vi "UT_Kolmogan.vi"() -> ()   [LabVIEW 2019, in "Kolmogan Library 1.lvlib"]
uses:
  Kolmogan Library 1.lvlib
panel:
  out "data out":string
  out "State":i32
  out "current time":timestamp
  out "Result":string
  in  "COGNEX Command":bool
  in  "IP:Port COGNEX Result":string="192.168.0.30"
  in  "IP:Port COGNEX Command":string="192.168.0.30:23"
  out "MS error out":errorcluster
  out "PL.FB error out":errorcluster
  in  "milliseconds to wait":u32=500
  in  "Continue Read":bool
  out "PL.FB":i64
  out "data":bool[](array[boolean])
  in  "RD_DRVMOTIONSTAT":bool
  in  "RD_POSITION_FEEDBACK":bool
  in  "KOLMOGAN指令":u8(ring) items=["0. 復歸", "1. 找原點", "2. 至起始位置", "3. 啟動相機", "4. 掃描拍攝", "SB"]
  out "Error Out":errorcluster
  in  "Error In":errorcluster
  in  "IP:Port":string="192.168.1.11:502"
  in  "Close API":bool
  in  "stop":bool
  in  "Connect PLC":bool
  # "Trigger+Call Motion"
  # "State machine (等待觸發燈號)\n1. 建立連線\n2. 復歸 [ SW(F), Camera(F) ]\n3. 找原點 (Home position found)\n4. 初始位置 (15)\n等待觸發\n>>相機\n>>掃描 (15)\n>>復歸 [ SW(F), Camera(F) ]\nError 重新建立連線"
  # "#588 959/1174 這邊要問Andy"
  # "#268 600/1174 State"
  # "1"
  # "2"
  # "3"
  # "Motion task reach position"
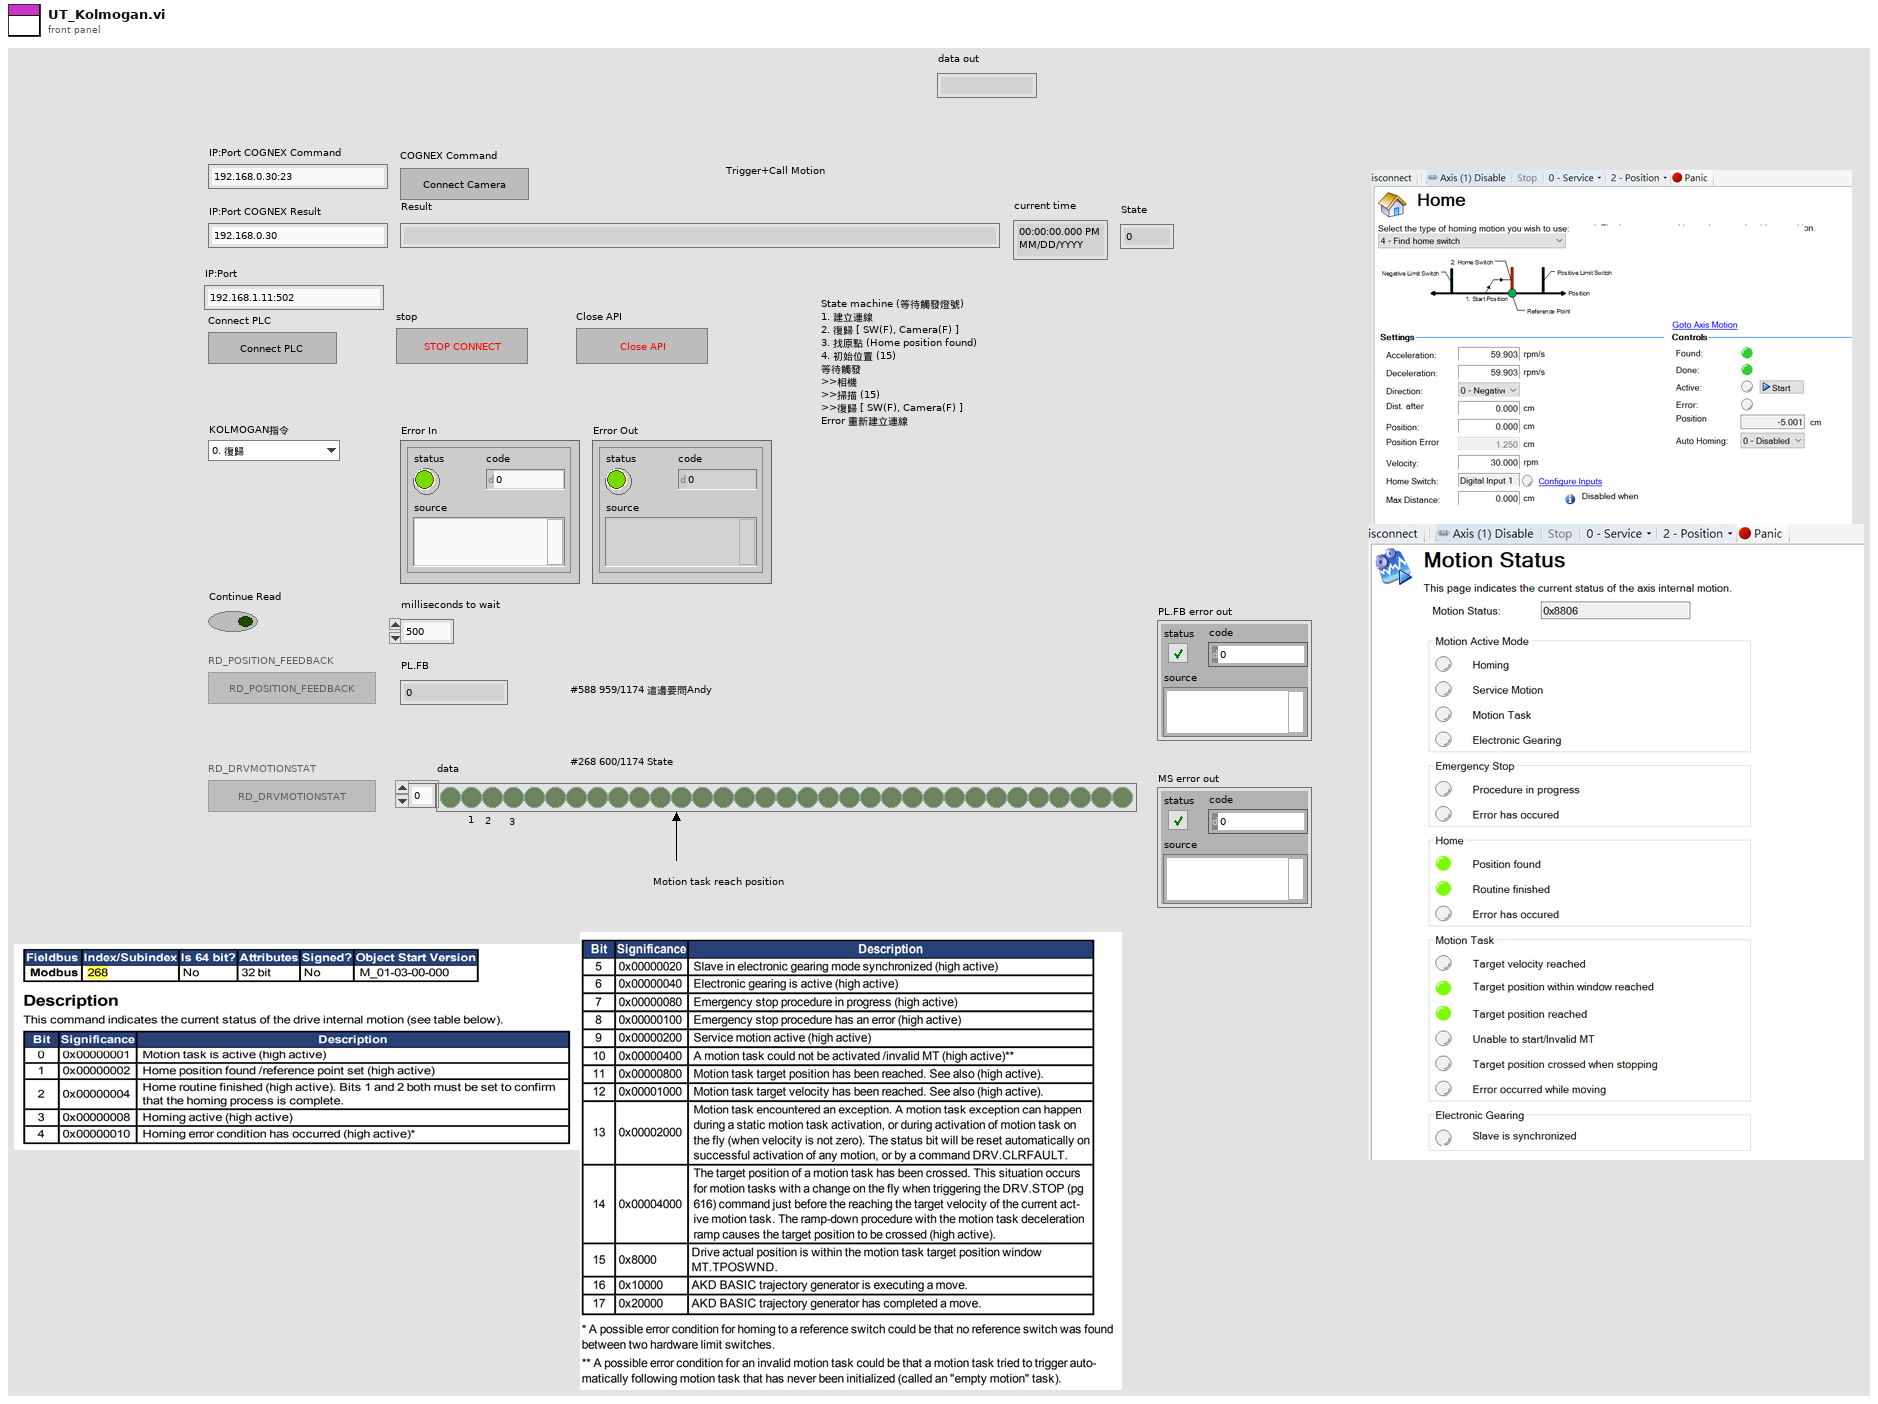
[diagram p1: front panel]
types:
  T1 = enum8{"Enabled", "Disabled", "Disabled and Grayed Out"}
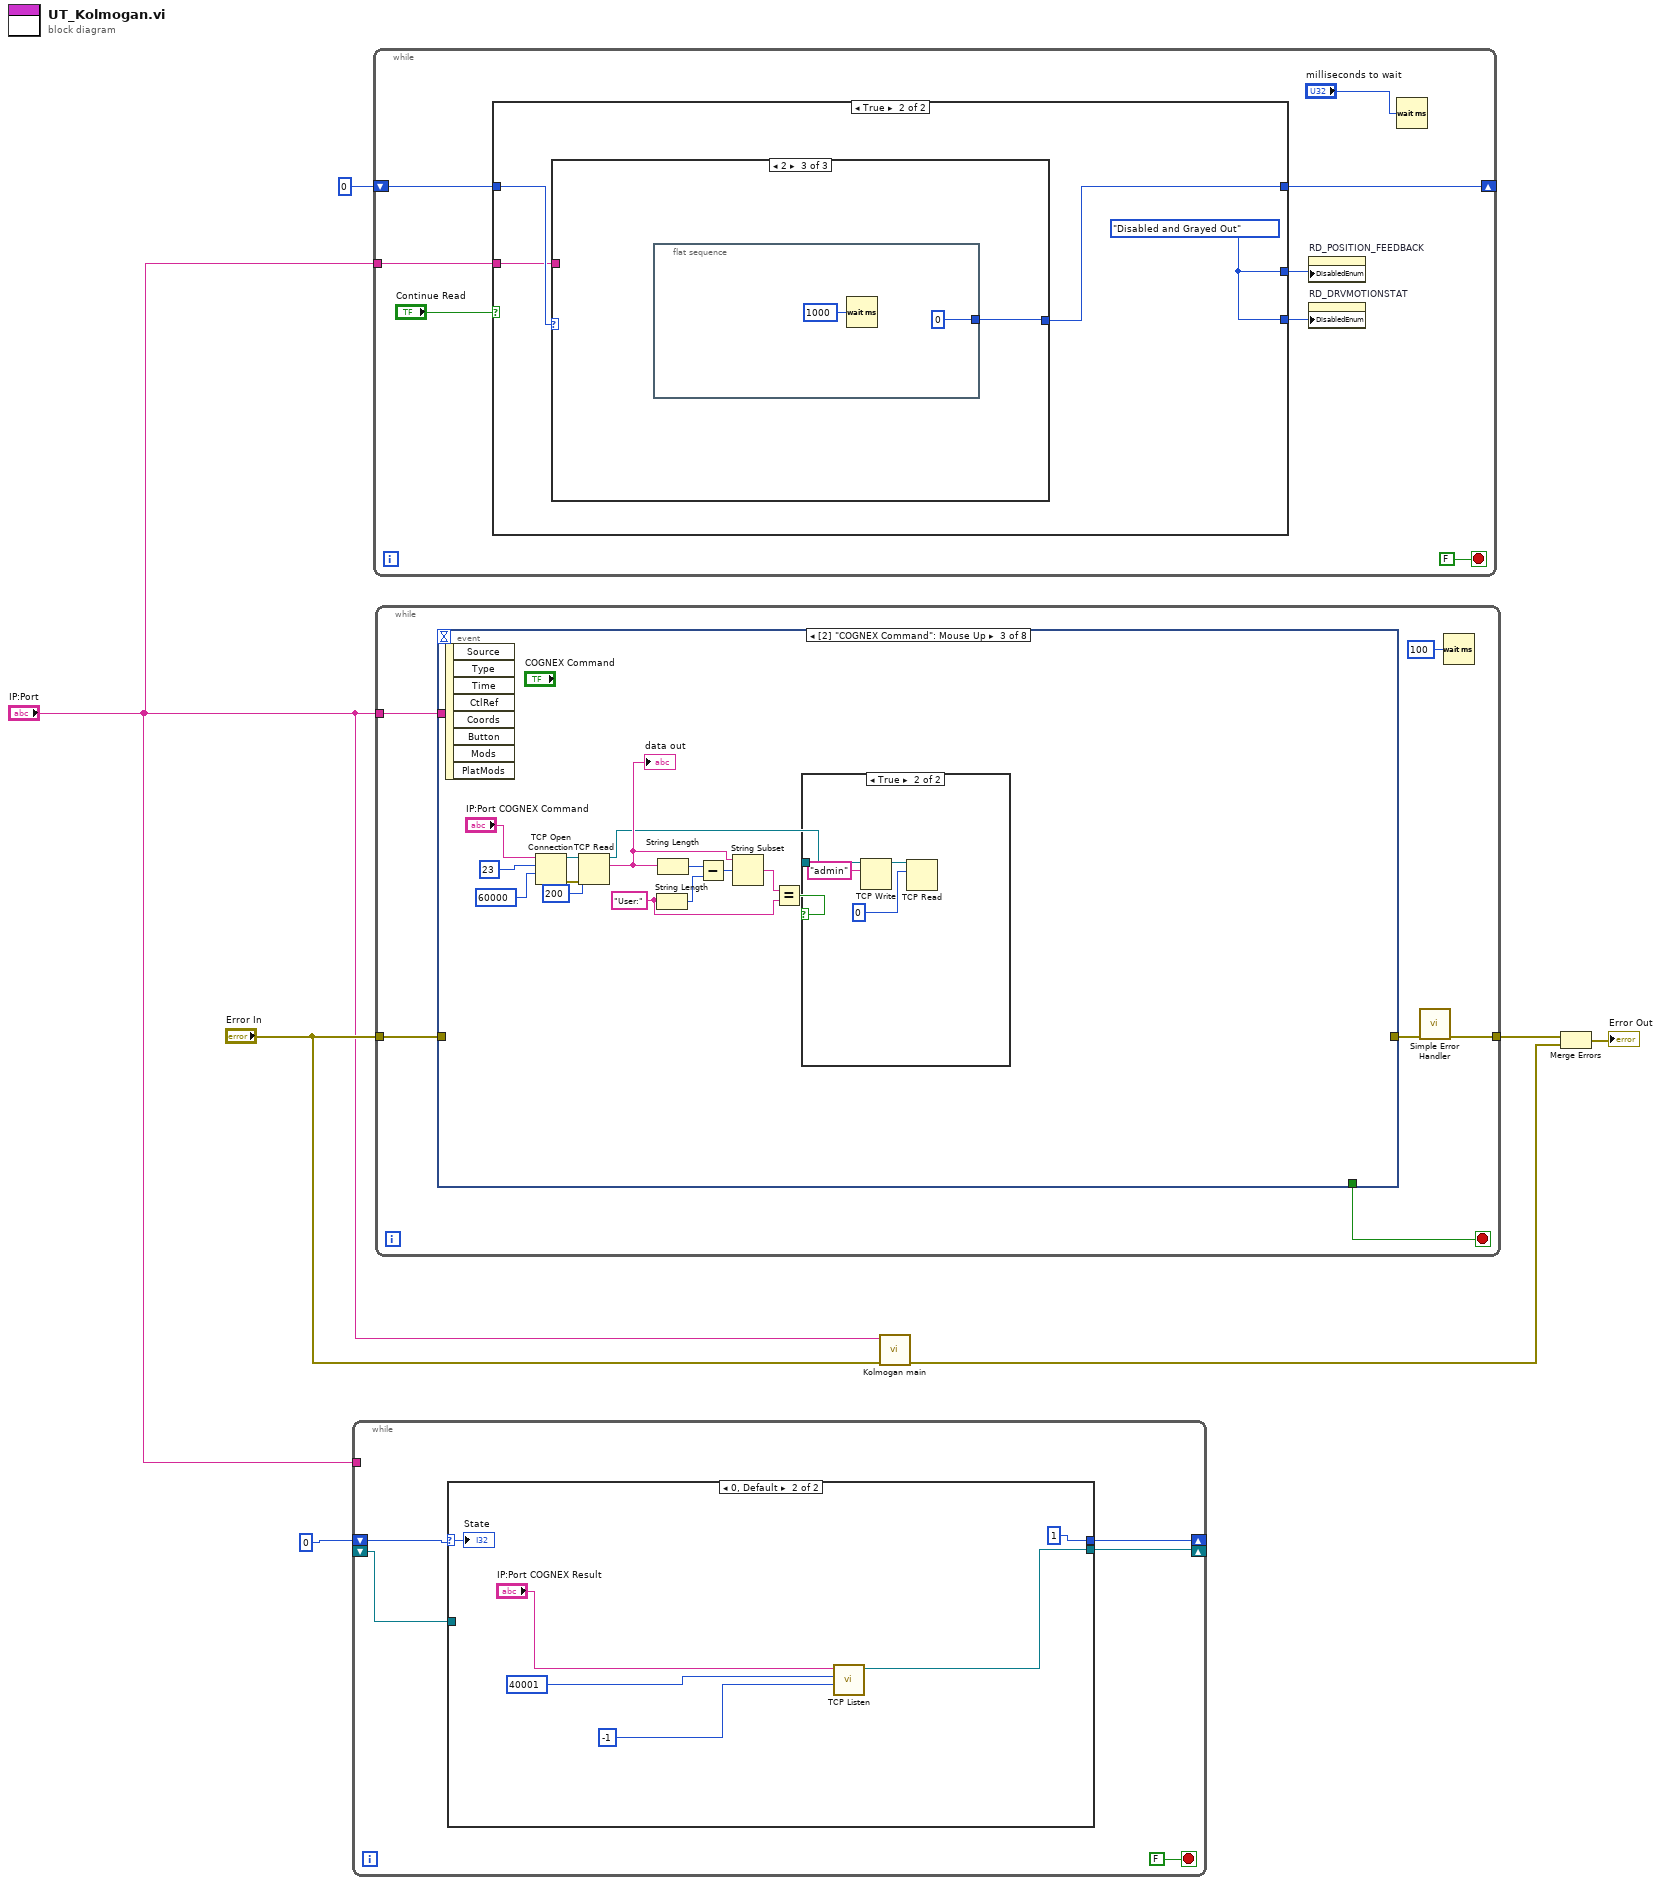
[diagram p0: block diagram]
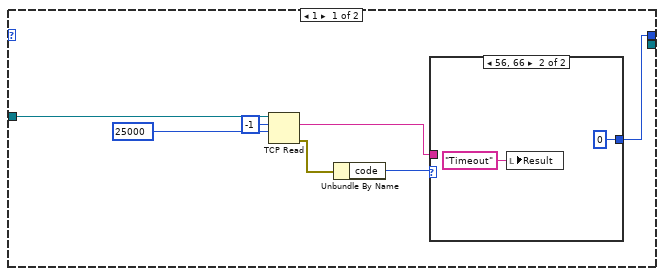
[diagram p2: hidden frame]
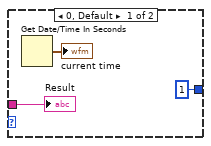
[diagram p3: hidden frame]
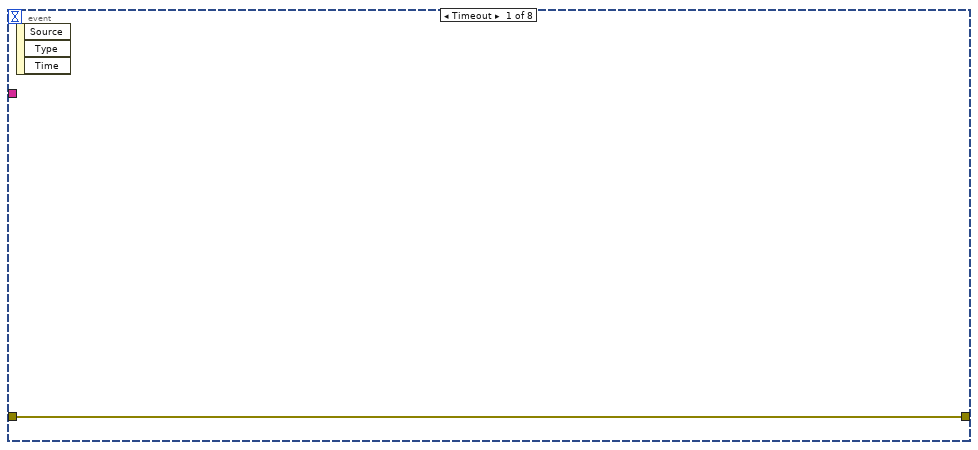
[diagram p4: hidden frame]
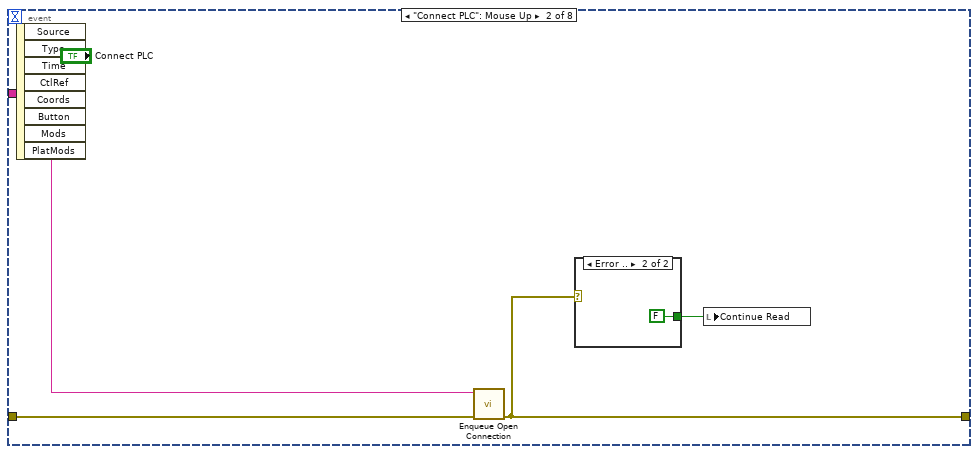
[diagram p5: hidden frame]
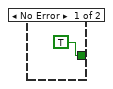
[diagram p6: hidden frame]
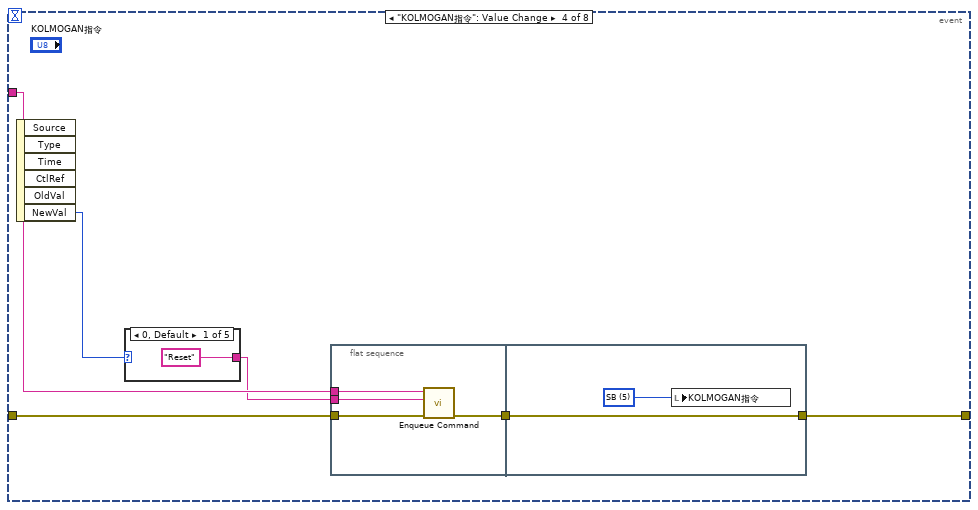
[diagram p8: hidden frame]
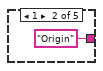
[diagram p9: hidden frame]
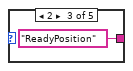
[diagram p10: hidden frame]
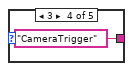
[diagram p11: hidden frame]
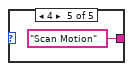
[diagram p12: hidden frame]
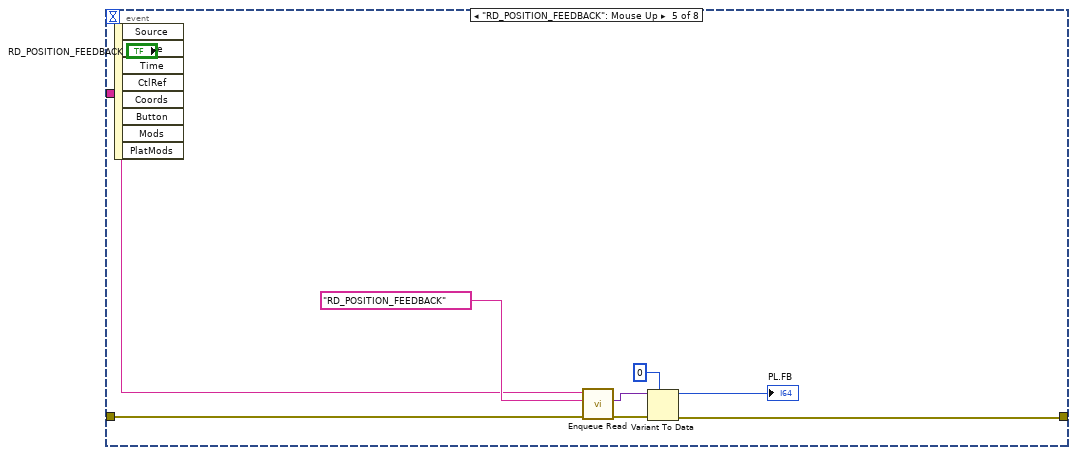
[diagram p13: hidden frame]
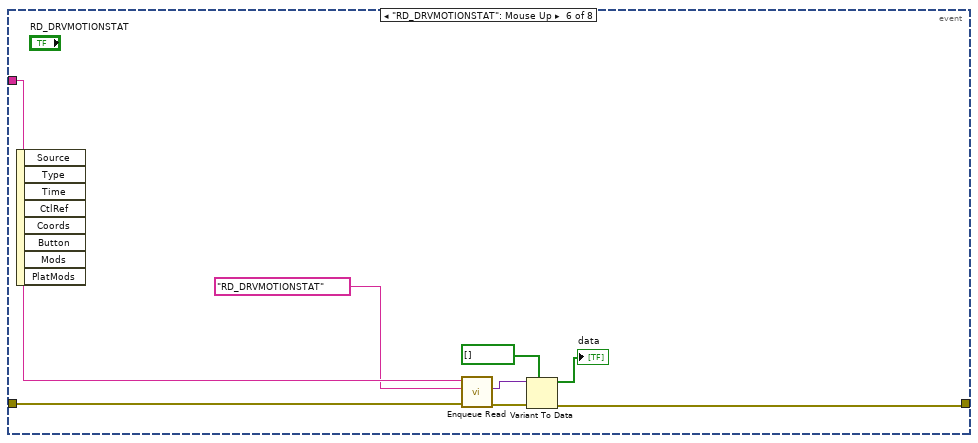
[diagram p14: hidden frame]
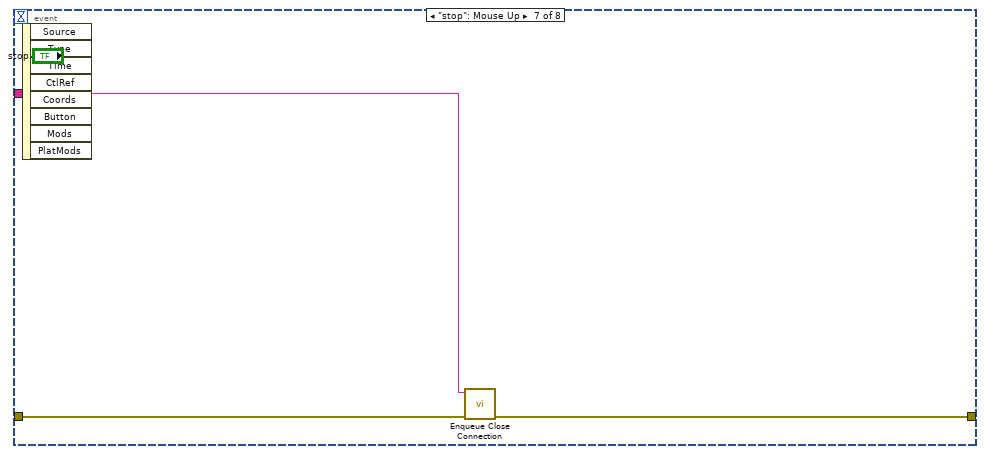
[diagram p15: hidden frame]
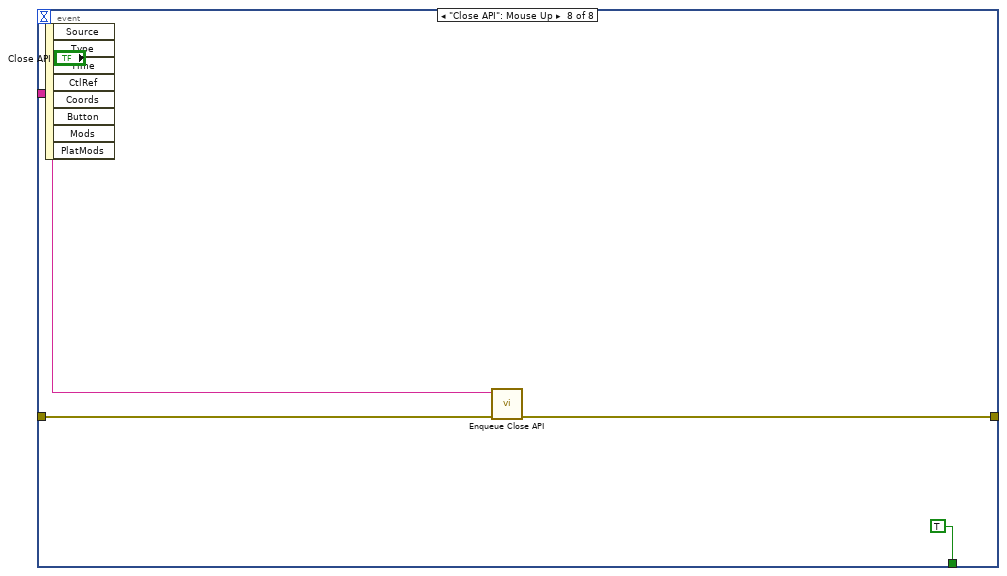
[diagram p16: hidden frame]
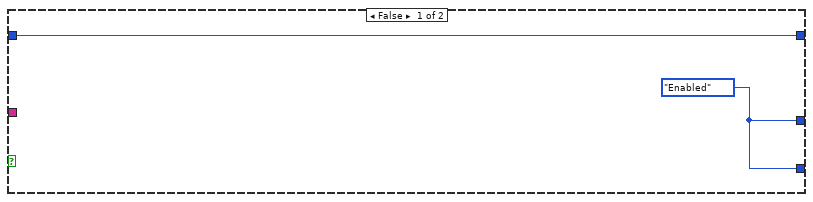
[diagram p17: hidden frame]
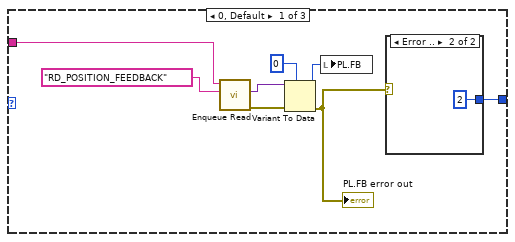
[diagram p18: hidden frame]
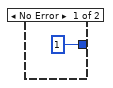
[diagram p19: hidden frame]
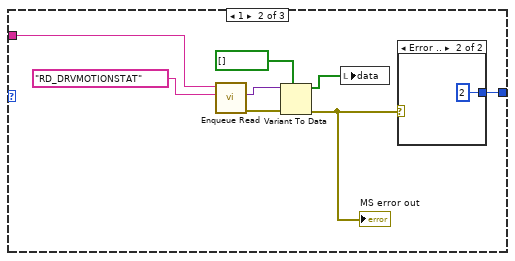
[diagram p20: hidden frame]
diagram:
  n1 = while {
    shift-right: [w11] -> _
    shift-left: _ -> [w8]
    shift-right: [w9] -> _
    shift-left: 0 ("timeout ms (wait forever: -1)") -> [w10]
    tunnel: "IP:Port" -> [_]
    stop <- FALSE stop-if-true
    n2 = case shown="0, Default" w10 {
      selector: w10 -> [_ w25]
      tunnel: [_ w27] -> w11
      tunnel: [w16 1 ("timeout ms (wait forever: -1)")] -> w9
      tunnel: w8 -> [w19 _]
      frame 1 {
        n3 = TCP Read(connection ID=w19, bytes to read=-1, 9:25000 ("timeout ms (25000)")) -> (data out=w13:string, error out=w15:errorcluster)  [unwired: 2 in, 1 out]
        n4 = Unbundle By Name(w15) -> ("code"=w14:i32)
        n5 = case shown="56, 66" w14 {
          tunnel: [1 ("timeout ms (wait forever: -1)") 0 ("timeout ms (wait forever: -1)")] -> w16
          tunnel: w13 -> [w21 _]
          frame 0, Default {
            n6 = Get Date/Time In Seconds() -> (seconds since 1Jan1904=→"current time":timestamp)
            "Result" <- w21
          }
          frame 56, 66 {
            n7 = local write "Result"("Timeout" ("Result")) -> ()
          }
        }
      }
      frame 0, Default {
        n8 = call <vilib>:"TCP Listen.vi"("timeout ms (wait forever: -1)"=-1, "port"=u16 40001, "service name"="IP:Port COGNEX Result") -> ("connection ID"=w27:refnum<k5>)  [unwired: 4 in, 4 out]
        "State" <- w25
      }
    }
  }
  n9 = while {
    tunnel: "IP:Port" -> [w34]
    shift-right: [w33] -> _
    shift-left: 0 -> [w32]
    stop <- FALSE stop-if-true
    n10 = case shown="True" "Continue Read" {
      tunnel: [w40 w44] -> w37
      tunnel: [w40 w44] -> w36
      tunnel: w32 -> [w39 w43]
      tunnel: w34 -> [_ w42]
      tunnel: [w39 w41] -> w33
      frame False {
        w40 = T1."Enabled" ("Disabled")
      }
      frame True {
        w44 = T1."Disabled and Grayed Out" ("Disabled")
        n11 = case shown="2" w43 {
          tunnel: w42 -> [w47 w57 _]
          tunnel: [w46 w56 w65] -> w41
          frame 0, Default {
            n12 = call "Enqueue Read.vi"("Message"="RD_POSITION_FEEDBACK", "Name"=w47) -> ("Error Out"=w50:errorcluster, "Data"=w51:variant)  [unwired: 8 in]
            n13 = Variant To Data(error in=w50, type=i64 0, Variant=w51) -> (data=w52:i64, error out=w45:errorcluster)
            "PL.FB error out" <- w45
            n14 = local write "PL.FB"(w52) -> ()
            n15 = case shown="Error .." w45 {
              tunnel: [1 2] -> w46
              frame No Error {
              }
              frame Error {
              }
            }
          }
          frame 1 {
            n16 = call "Enqueue Read.vi"("Message"="RD_DRVMOTIONSTAT", "Name"=w57) -> ("Error Out"=w60:errorcluster, "Data"=w61:variant)  [unwired: 8 in]
            n17 = Variant To Data(error in=w60, type=bool[] [] ("appended array"), Variant=w61) -> (data=w62:bool[], error out=w55:errorcluster)
            "MS error out" <- w55
            n18 = local write "data"(w62) -> ()
            n19 = case shown="Error .." w55 {
              tunnel: [0 2] -> w56
              frame No Error {
              }
              frame Error {
              }
            }
          }
          frame 2 {
            n20 = flat-sequence {
              tunnel: [0] -> w65
              frame #0 {
                n21 = Wait (ms)(milliseconds to wait=u32 1000) -> ()  [unwired: 1 out]
              }
            }
          }
        }
      }
    }
    n22 = property on="RD_POSITION_FEEDBACK" class="Bool (strict)"("DisabledEnum"=w37) -> ()  [unwired: 2 in, 2 out]
    n23 = property on="RD_DRVMOTIONSTAT" class="Bool (strict)"("DisabledEnum"=w36) -> ()  [unwired: 2 in, 2 out]
    n24 = Wait (ms)(milliseconds to wait="milliseconds to wait") -> ()  [unwired: 1 out]
  }
  n25 = while {
    tunnel: "IP:Port" -> [w73]
    tunnel: "Error In" -> [w72]
    tunnel: [w70] -> w6
    stop <- w69 stop-if-true
    n26 = event shown="[2] \"COGNEX Command\": Mouse Up" {
      selector: _ -> [_ _ _ _ _ _ _ _]
      dyn-events: _ -> [_ _ _ _ _ _ _ _]
      timeout: _ -> [_ _ _ _ _ _ _ _]
      tunnel: w73 -> [_ w77 _ w103 w119 w131 w133 w137]
      tunnel: w72 -> [w74 w78 _ w102 w120 w130 w134 w138]
      tunnel: [w74 w76 _ w101 w117 w126 w132 w136] -> w71
      tunnel: [_ _ _ _ _ _ _ TRUE] -> w69
      event Timeout {
        n27 = event-data() -> ()  [unwired: 1 in, 3 out]
      }
      event "Connect PLC": Mouse Up {
        n28 = event-data() -> ()  [unwired: 1 in, 8 out]
        n29 = call "Enqueue Open Connection.vi"("Error In"=w78, "Name"=w77) -> ("Error Out"=w76:errorcluster)  [unwired: 9 in]
        n30 = case shown="Error .." w76 {
          tunnel: [TRUE ("Continue Read") FALSE ("Continue Read")] -> w75
          frame No Error {
          }
          frame Error {
          }
        }
        n31 = local write "Continue Read"(w75) -> ()
      }
      event "COGNEX Command": Mouse Up {
        w83 = "User:" ("string")
        n32 = event-data() -> ()  [unwired: 1 in, 8 out]
        n33 = TCP Open Connection(address="IP:Port COGNEX Command", remote port or service name=u16 23, timeout ms (60000)=60000) -> (connection ID=w90:refnum<k5>, error out=w91:errorcluster)  [unwired: 2 in]
        n34 = TCP Read(connection ID=w90, bytes to read=200, error in (no error)=w91) -> (connection ID out=w81:refnum<k5>, data out=w85:string)  [unwired: 2 in, 1 out]
        "data out" <- w85
        n35 = String Length(string=w83) -> (length=w88:i32)
        n36 = String Length(string=w85) -> (length=w89:i32)
        n37 = Subtract(x=w89, y=w88) -> (x-y=w87:i32)
        n38 = String Subset(string=w85, offset (0)=w87) -> (substring=w84:string)  [unwired: 1 in]
        n39 = Equal?(x=w84, y=w83) -> (x = y?=w82:bool)
        n40 = case shown="True" w82 {
          tunnel: w81 -> [_ w98]
          frame False {
          }
          frame True {
            n41 = TCP Write(connection ID=w98, data in="admin") -> (connection ID out=w96:refnum<k5>)  [unwired: 2 in, 2 out]
            n42 = TCP Read(connection ID=w96, bytes to read=0) -> ()  [unwired: 3 in, 3 out]
          }
        }
      }
      event "KOLMOGAN指令": Value Change {
        n43 = event-data() -> ("NewVal"=w104:u8)  [unwired: 1 in, 5 out]
        n44 = case shown="0, Default" w104 {
          tunnel: ["Reset" "Origin" "ReadyPosition" "CameraTrigger" "Scan Motion"] -> w100
          frame 0, Default {
          }
          frame 1 {
          }
          frame 2 {
          }
          frame 3 {
          }
          frame 4 {
          }
        }
        n45 = flat-sequence {
          tunnel: w103 -> [w108]
          tunnel: w102 -> [w107]
          tunnel: w100 -> [w105]
          tunnel: [w106] -> w99
          tunnel: [w110] -> w101
          tunnel: w99 -> [w110]
          frame #0 {
            n46 = call "Enqueue Command.vi"("Error In"=w107, "Message"=w105, "Name"=w108) -> ("Error Out"=w106:errorcluster)  [unwired: 8 in]
          }
          frame #1 {
            w109 = u8 5 items=["0. 復歸", "1. 找原點", "2. 至起始位置", "3. 啟動相機", "4. 掃描拍攝", "SB"] ("KOLMOGAN指令")
            n47 = local write "KOLMOGAN指令"(w109) -> ()
          }
        }
      }
      event "RD_POSITION_FEEDBACK": Mouse Up {
        n48 = event-data() -> ()  [unwired: 1 in, 8 out]
        n49 = call "Enqueue Read.vi"("Error In"=w120, "Message"="RD_POSITION_FEEDBACK", "Name"=w119) -> ("Error Out"=w121:errorcluster, "Data"=w122:variant)  [unwired: 7 in]
        n50 = Variant To Data(error in=w121, type=i64 0, Variant=w122) -> (data=→"PL.FB":i64, error out=w117:errorcluster)
      }
      event "RD_DRVMOTIONSTAT": Mouse Up {
        n51 = event-data() -> ()  [unwired: 1 in, 8 out]
        n52 = call "Enqueue Read.vi"("Error In"=w130, "Message"="RD_DRVMOTIONSTAT", "Name"=w131) -> ("Error Out"=w127:errorcluster, "Data"=w128:variant)  [unwired: 7 in]
        n53 = Variant To Data(error in=w127, type=bool[] [] ("appended array"), Variant=w128) -> (data=→"data":bool[], error out=w126:errorcluster)
      }
      event "stop": Mouse Up {
        n54 = event-data() -> ()  [unwired: 1 in, 8 out]
        n55 = call "Enqueue Close Connection.vi"("Error In"=w134, "Name"=w133) -> ("Error Out"=w132:errorcluster)  [unwired: 9 in]
      }
      event "Close API": Mouse Up {
        n56 = event-data() -> ()  [unwired: 1 in, 8 out]
        n57 = call "Enqueue Close API.vi"("Error In"=w138, "Name"=w137) -> ("Error Out"=w136:errorcluster)  [unwired: 9 in]
      }
    }
    n58 = call <vilib>:"Simple Error Handler.vi"("error in (no error)"=w71) -> ("error out"=w70:errorcluster)  [unwired: 4 in, 4 out]
    n59 = Wait (ms)(milliseconds to wait=u32 100) -> ()  [unwired: 1 out]
  }
  n60 = call "Kolmogan main.vi"("Error In"="Error In", "Name"="IP:Port") -> ("Error Out"=w5:errorcluster)  [unwired: 9 in]
  n61 = Merge Errors(w6, w5) -> (→"Error Out":errorcluster)
